vi "GetAzCamToolParameter.vi"(0 "Parameter":string) -> (1 "Error":bool, 2 "Value":string)   [LabVIEW 2014]
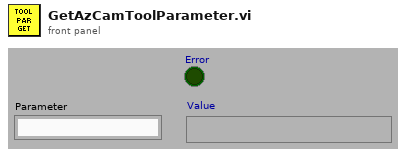
[diagram p1: front panel]
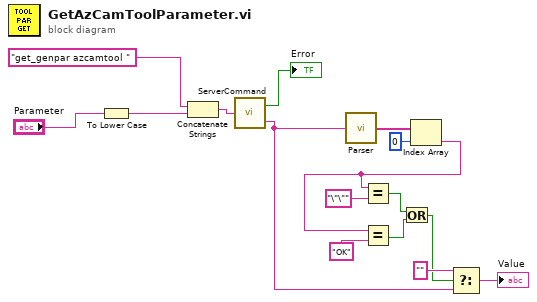
[diagram p0: block diagram]
diagram:
  n1 = To Lower Case(string="Parameter") -> (all lower case string=w1:string)
  n2 = Concatenate Strings("get_genpar azcamtool " ("Attribute"), w1) -> (w2:string)
  n3 = call "ServerCommand.vi"("Command"=w2) -> ("Error"=→"Error":bool, "Reply"=w10:string)
  n4 = call "Parser.vi"("string"=w10) -> ("Out Strings"=w14:string[])
  n5 = Index Array(array=w14, index=0) -> (element=w9:string)
  n6 = Equal?(x=w9, y="\"\"") -> (x = y?=w7:bool)
  n7 = Equal?(x=w9, y="OK") -> (x = y?=w6:bool)
  n8 = Or(x=w7, y=w6) -> (x .or. y?=w5:bool)
  n9 = Select(t="", s=w5, f=w10) -> (s? t:f=→"Value":string)
